vi "test - read from INI String.vi"(8 "error in (no error)":errorcluster, 11 "TestCase in":refnum<class "csm-ini-variable-addon.lvclass">) -> (0 "error out":errorcluster, 3 "TestCase out":refnum<class "csm-ini-variable-addon.lvclass">)   [LabVIEW 2017, in "csm-ini-variable-addon.lvclass"]
uses:
  csm-ini-variable-addon.lvclass
  <vilib>/addons/_JKI Toolkits/VI Tester/TestCase.llb/TestCase.lvclass
  INI-Static-Variable-Support/INI-Static-Variable-Support.lvlib
  <userlib>/_NEVSTOP/Communicable State Machine(CSM)/addons/API-String-Arugments-Support/API String Arguments Support.lvlib
  C:/Program Files (x86)/National Instruments/LabVIEW 2017/vi.lib/addons/_JKI Toolkits/VI Tester/TestCase.llb/TestCase.lvclass
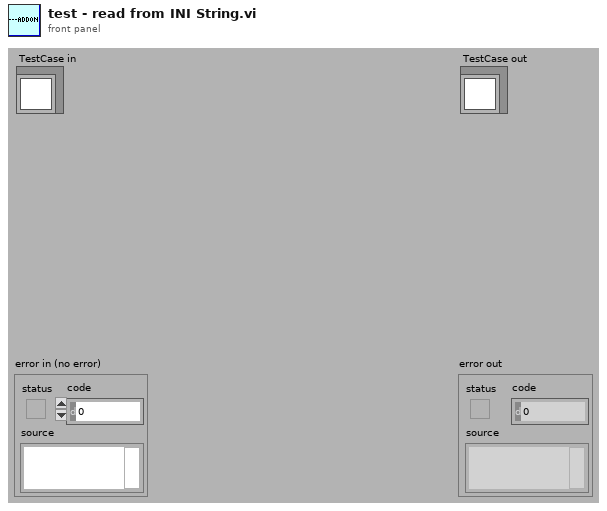
[diagram p1: front panel]
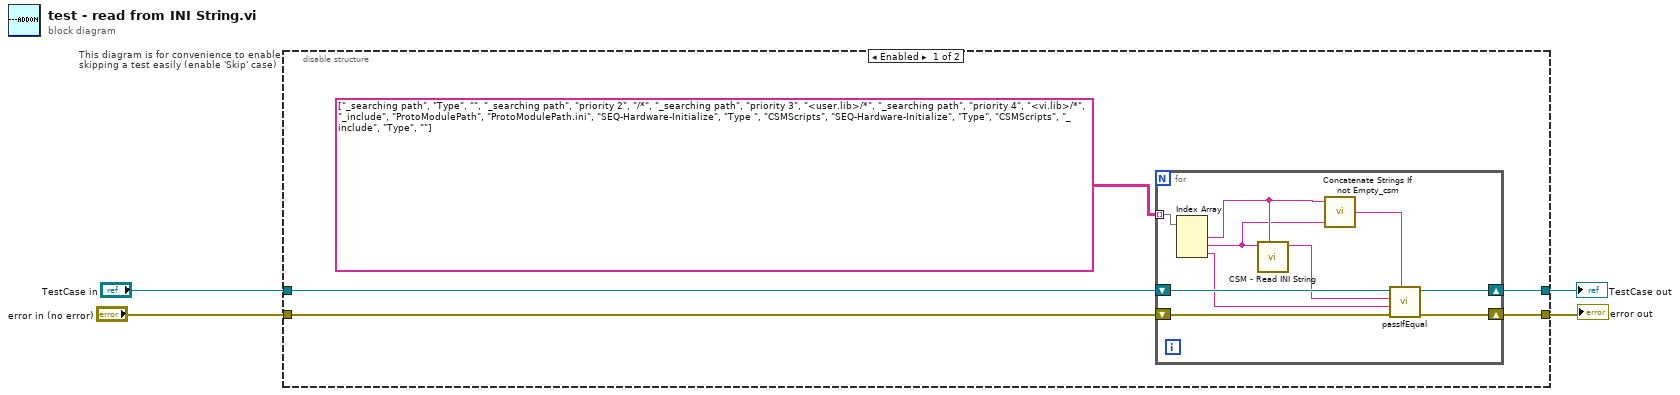
[diagram p0: block diagram]
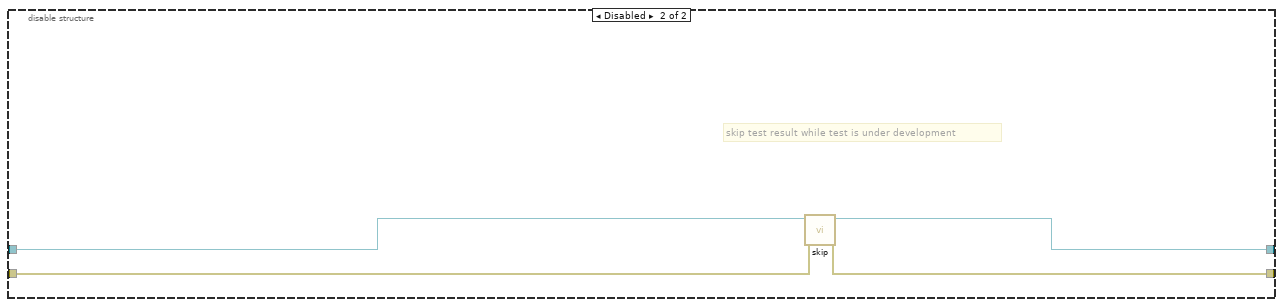
[diagram p2: hidden frame]
diagram:
  n1 = disable-structure "This diagram is for convenience to enable skipping a test easily (enable 'Skip' case)" shown="Enabled" {
    disable-tunnel: "TestCase in" -> [w6 w23]
    disable-tunnel: [w9 w21] -> w1
    disable-tunnel: [w8 w22] -> w3
    disable-tunnel: "error in (no error)" -> [w7 w20]
    frame Enabled {
      n2 = for {
        shift-right: [w18] -> w8
        shift-left: w7 -> [w17]
        shift-right: [w19] -> w9
        shift-left: w6 -> [w16]
        tunnel: string[][] [["_searching path", "Type", ""], ["_searching path", "priority 2", "/*"], ["_searching path", "priority 3", "<user.lib>/*"], ["_searching path", "priority 4", "<vi.lib>/*"], ["_include", "ProtoModulePath", "ProtoModulePath.ini"], ["SEQ-Hardware-Initialize", "Type ", "CSMScripts"], ["SEQ-Hardware-Initialize", "Type", "CSMScripts"], ["_include", "Type", ""]] -> [w14] mode=indexing
        n3 = Index Array(array=w14) -> (element #1=w11:string, element #2=w10:string, element #3=w13:string)  [unwired: 3 in]
        n4 = call "CSM - Read INI String.vi"("Section Name(\"\" as Default)"=w11, "String in"=w10) -> ("String out"=w15:string)  [unwired: 5 in, 2 out]
        n5 = call <userlib>:"Concatenate Strings If not Empty_csm.vi"("String"=w10, "prefix"=w11) -> ("result"=w12:string)  [unwired: 3 in]
        n6 = call-dynamic "passIfEqual.vi"("custom report message (\"\")"=w12, "error in (no error)"=w17, "y"=w13, "x"=w15, "TestCase in"=w16) -> ("error out"=w18:errorcluster, "TestCase out"=w19:refnum<class "csm-ini-variable-addon.lvclass">)  [unwired: 5 in]
      }
    }
    frame Disabled {
      # "skip test result while test is under development"
      n7 = call <vilib>:"skip.vi"("error in (no error)"=w20, "TestCase in"=w23) -> ("error out"=w22:errorcluster, "TestCase out"=w21:refnum<class "csm-ini-variable-addon.lvclass">)  [unwired: 8 in]
    }
  }
  "error out" <- w3
  "TestCase out" <- w1
